vi "SQL Build Select_Condition Query.vi"(8 "error in (no error)":errorcluster, 9 "condition":string, 10 "columns":string[](array[string]), 11 "table":string) -> (0 "error out":errorcluster, 3 "select query":string)   [LabVIEW 2011]
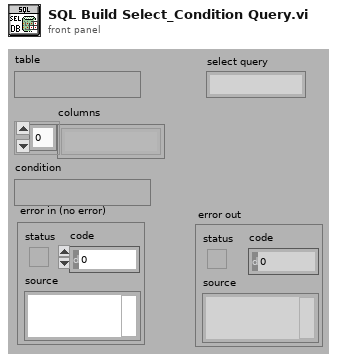
[diagram p1: front panel]
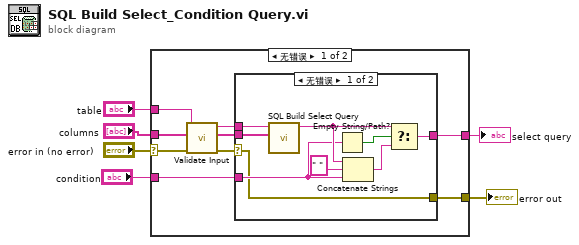
[diagram p0: block diagram]
diagram:
  n1 = case shown="无错误" "error in (no error)" {
    selector: "error in (no error)" -> [w9 w26]
    tunnel: "table" -> [w15 _]
    tunnel: "columns" -> [w11 _]
    tunnel: "condition" -> [w10 _]
    tunnel: [w8 _] -> w2
    tunnel: [w7 w26] -> w1
    frame No Error {
      n2 = call "Validate Input.vi"("error in (no error)"=w9, "columns"=w11, "table"=w15) -> ("error out"=w12:errorcluster, "columns out"=w14:string[], "table out"=w13:string)  [unwired: 6 in]
      n3 = case shown="无错误" w12 {
        selector: w12 -> [w16 w25]
        tunnel: w14 -> [w18 _]
        tunnel: w13 -> [w24 _]
        tunnel: w10 -> [w19 _]
        tunnel: [w17 _] -> w8
        tunnel: [w16 w25] -> w7
        frame No Error {
          n4 = call "SQL Build Select Query.vi"("columns"=w18, "table name"=w24) -> ("select query"=w22:string)  [unwired: 9 in]
          n5 = Empty String/Path?(string/path=w19) -> (empty?=w23:bool)
          n6 = Concatenate Strings(w22, " " ("Substring"), w19) -> (w21:string)
          n7 = Select(t=w22, s=w23, f=w21) -> (s? t:f=w17:string)
        }
        frame Error {
        }
      }
    }
    frame Error {
    }
  }
  "select query" <- w2
  "error out" <- w1
